vi "PhotonCamera_TakeInputSnapshot.vi"(11 "CameraName":string) -> ()   [LabVIEW 2019, in "PhotonVisionLib.lvlib"]
doc: "Request the camera to save a new image file from the input camera stream with overlays. Images take up space in the filesystem of the PhotonCamera. Calling it frequently will fill up disk space and eventually cause the system to stop working. Clear out images in /opt/photonvision/photonvision_config/imgSaves frequently to prevent issues.\n\nInputs:\n - cameraName -- The nickname of the camera (found in the PhotonVision UI).\n\nOutputs:\n - >none<"
uses:
  PhotonVisionLib.lvlib
  <vilib>/Rock Robotics/Network Tables/NT Read Number.vi
  <vilib>/Rock Robotics/Network Tables/NT Write Number.vi
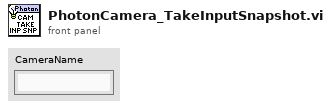
[diagram p1: front panel]
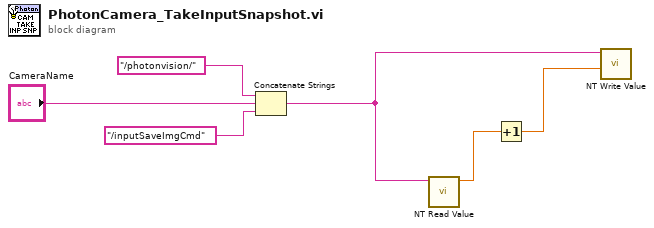
[diagram p0: block diagram]
diagram:
  n1 = Concatenate Strings("/photonvision/", "CameraName", "/inputSaveImgCmd") -> (w3:string)
  n2 = call-poly <vilib>:"NT Read Value.vi"("Name"=w3) -> ("Numeric"=w2:dbl)  [unwired: 9 in, 1 out]
  n3 = Increment(x=w2) -> (x+1=w1:dbl)
  n4 = call-poly <vilib>:"NT Write Value.vi"("Numeric"=w1, "Name"=w3) -> ()  [unwired: 9 in, 1 out]
